vi "20220114_04.vi"(1 "Function":T1, 2 "Input":dbl) -> (0 "Output":dbl)   [LabVIEW 2019]
uses:
  20220114_04_Function.ctl
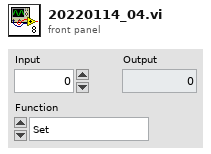
[diagram p1: front panel]
types:
  T1 = typedef "20220114_04_Function.ctl" = enum16{"Set", "Get", "Reset"}
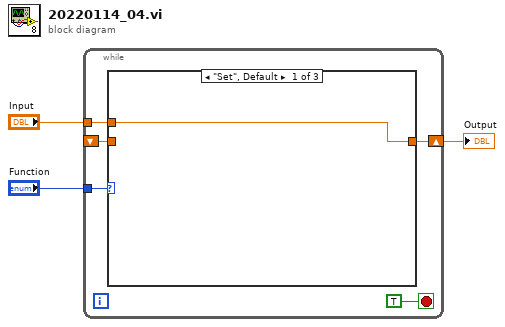
[diagram p0: block diagram]
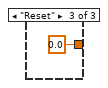
[diagram p3: hidden frame]
diagram:
  n1 = while {
    shift-right: [w6] -> w1
    shift-left: _ -> [w4]
    tunnel: "Function" -> [w7]
    tunnel: "Input" -> [w5]
    stop <- TRUE stop-if-true
    n2 = case shown="\"Set\", Default" w7 {
      tunnel: [w9 w10 0.0 ("Input")] -> w6
      tunnel: w5 -> [w9 _ _]
      tunnel: w4 -> [_ w10 _]
      frame "Set", Default {
      }
      frame "Get" {
      }
      frame "Reset" {
      }
    }
  }
  "Output" <- w1
